vi "Send Message To Execution Engine.vi"(0 "Message":string, 5 "Message Type":i32(ring) items=["Info", "Warning", "Error", "Action"], 11 "error in (no error)":errorcluster) -> (15 "error out":errorcluster)   [LabVIEW 2023, in "RFCalAndFixtureCharact.Common.lvlib"]
uses:
  RFCalAndFixtureCharact.Common.lvlib
  C:/srd-semi-rfcal-software/AuxTools/STSRFFixtureCharactUtility/Source/Code Modules/Dependencies/NationalInstruments.RFCalibration.ExecutionEngine.dll
  Dependencies/NationalInstruments.RFCalibration.ExecutionEngine.dll
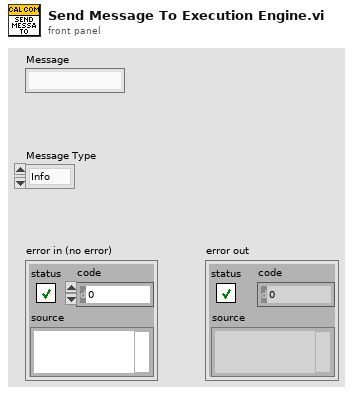
[diagram p1: front panel]
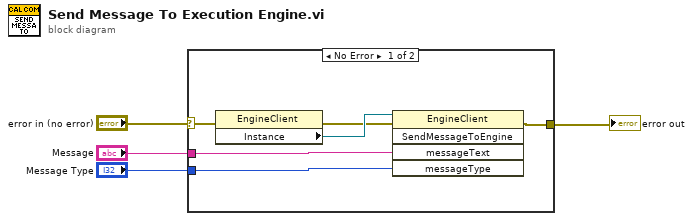
[diagram p0: block diagram]
diagram:
  n1 = case shown="No Error" "error in (no error)" {
    selector: "error in (no error)" -> [w6 w11]
    tunnel: [w10 w11] -> w3
    tunnel: "Message" -> [w9 _]
    tunnel: "Message Type" -> [w5 _]
    frame No Error {
      n2 = property class="EngineClient"(error in=w6) -> (error out=w7:errorcluster, "Instance"=w8:refnum<k24>)  [unwired: 1 in, 1 out]
      n3 = invoke class="EngineClient" method="SendMessageToEngine"(reference=w8, error in=w7, "messageText"=w9, "messageType"=w5) -> (error out=w10:errorcluster)  [unwired: 1 in, 4 out]
    }
    frame Error {
    }
  }
  "error out" <- w3
